vi "GetSystemDataResults.vi"(6 "argument":i32, 8 "error in (no error)":errorcluster, 9 "system data signal":u32(ring)=74 items=["DataCollectionSampleIndex"=161, "DataCollectionSampleTime"=149, "DataCollectionStatus"=255, "DriveModbusMasterInputBits"=354, "DriveModbusMasterInputWords"=352, "DriveModbusMasterOutputBits"=355, "DriveModbusMasterOutputStatusBits"=356, "DriveModbusMasterOutputStatusWords"=357, "DriveModbusMasterOutputWords"=353, "EstimatedProcessorUsage"=236, "FieldbusActiveConnections"=287, "FieldbusConnected"=284, "FieldbusErrorCode"=285, "FieldbusErrorLocation"=286, "FieldbusInactiveConnections"=288, "FieldbusInputs"=340, "FieldbusOutputs"=341, "GlobalVariable"=74, "LibraryCommand"=148, "ModbusMasterInputBits"=344, "ModbusMasterInputWords"=342, "ModbusMasterOutputBits"=345, "ModbusMasterOutputStatusBits"=346, "ModbusMasterOutputStatusWords"=347, "ModbusMasterOutputWords"=343, "ModbusSlaveInputBits"=350, "ModbusSlaveInputWords"=348, "ModbusSlaveOutputBits"=351, "ModbusSlaveOutputWords"=349, "PCModbusMasterConnected"=170, "PCModbusMasterErrorCode"=174, "PCModbusMasterErrorLocation"=176, "PCModbusSlaveConnected"=171, "PCModbusSlaveErrorCode"=175, "PCModbusSlaveErrorLocation"=177, "PLCBool"=211, "PLCByte"=212, "PLCDint"=217, "PLCDword"=214, "PLCInt"=216, "PLCLreal"=222, "PLCReal"=221, "PLCSint"=215, "PLCUdint"=220, "PLCUint"=219, "PLCUsint"=218, "PLCWord"=213, "SafeZoneActiveMask"=321, "SafeZoneViolationMask"=289, "ScopetrigID"=209, "SignalLogState"=270, "StopWatchTimer"=197, "SystemParameter"=379, "Timer"=56, "TimerPerformance"=57, "VirtualBinaryInput"=51, "VirtualBinaryOutput"=52, "VirtualRegisterInput"=53, "VirtualRegisterOutput"=54, "ZYGOPosition1"=164, "ZYGOPosition2"=165, "ZYGOPosition3"=166, "ZYGOPosition4"=167], 10 "Data In":refnum<k24>, 11 "controller in":refnum<k24>) -> (0 "error out":errorcluster, 1 "SystemData":dbl[](array[numeric]), 2 "Data Out":refnum<k24>, 3 "controller out":refnum<k24>)   [LabVIEW 2016, in "Aerotech VIs.lvlib"]
uses:
  Aerotech VIs.lvlib
  C:/Users/HEP Gantry/Documents/Assembly/V4/Drivers/Aerotech A3200/Bin/Aerotech.A3200.dll
  V4/Drivers/Aerotech A3200/Bin/Aerotech.A3200.dll
  C:/Users/HEP Gantry/Documents/Assembly/V4/Drivers/Aerotech A3200/Bin/Aerotech.A3200.LabVIEW.dll
  V4/Drivers/Aerotech A3200/Bin/Aerotech.A3200.LabVIEW.dll
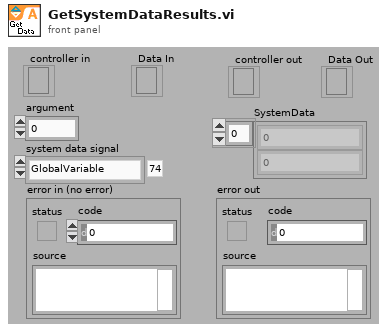
[diagram p1: front panel]
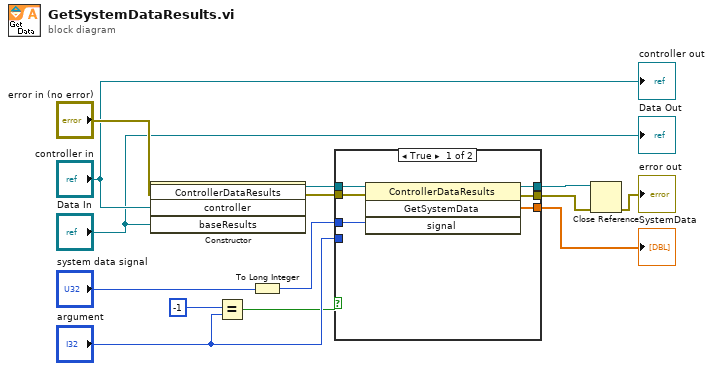
[diagram p0: block diagram]
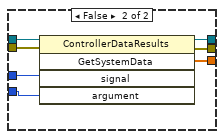
[diagram p2: hidden frame]
diagram:
  n1 = constructor class="ControllerDataResults"(error in="error in (no error)", "controller"="controller in", "baseResults"="Data In") -> (reference out=w14:refnum<k24>, error out=w13:errorcluster)  [unwired: 2 in, 3 out]
  n2 = Equal?(x=-1, y="argument") -> (x = y?=w5:bool)
  n3 = To Long Integer(number="system data signal") -> (32bit integer=w4:i32)
  n4 = case shown="True" w5 {
    tunnel: w4 -> [w15 w22]
    tunnel: [w20 w27] -> w3
    tunnel: [w19 w26] -> w2
    tunnel: w14 -> [w18 w25]
    tunnel: w13 -> [w17 w24]
    tunnel: "argument" -> [_ w21]
    tunnel: [w16 w23] -> w12
    frame True {
      n5 = invoke class="ControllerDataResults" method="GetSystemData"(reference=w18, error in=w17, "signal"=w15) -> (reference out=w19:refnum<k24>, error out=w20:errorcluster, "GetSystemData"=w16:dbl[])  [unwired: 1 in, 1 out]
    }
    frame False {
      n6 = invoke class="ControllerDataResults" method="GetSystemData"(reference=w25, error in=w24, "signal"=w22, "argument"=w21) -> (reference out=w26:refnum<k24>, error out=w27:errorcluster, "GetSystemData"=w23:dbl[])  [unwired: 1 in, 2 out]
    }
  }
  "SystemData" <- w12
  n7 = Close Reference(reference=w2, error in (no error)=w3) -> (error out=→"error out":errorcluster)
  "controller out" <- "controller in"
  "Data Out" <- "Data In"
